vi "irrad calc lumens.vi"(8 "error in (no error)":errorcluster, 10 "IRRAD Input Parameters":T1, 11 "Color Parameters in":T2) -> (0 "error out":errorcluster, 2 "IRRAD Input Parameters out":T1, 3 "Color Parameters out":T2)   [LabVIEW 2013, in "AvaSpec.lvlib" / "AVSirrad_support.lvlib"]
uses:
  AVSirrad_support.lvlib
  Acquisition/AvaSpec Color Parameters.ctl
  Acquisition/Sphere Indicator.ctl
  IRRAD input parameters.ctl
  Libraries/IRRAD-DLL/AVSirrad.lvlib
  AvaSpec.lvlib
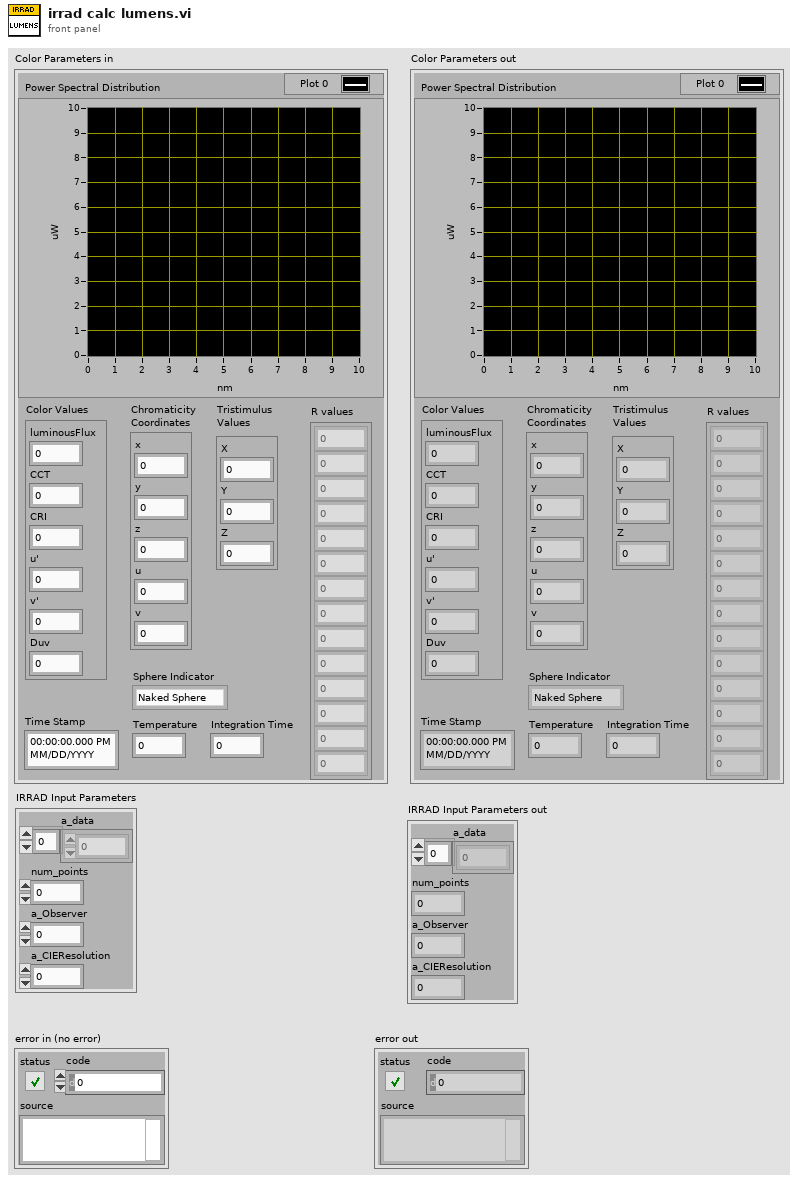
[diagram p1: front panel]
types:
  T1 = typedef "IRRAD input parameters.ctl" = cluster{"a_data":dbl[], "num_points":i32, "a_Observer":u8, "a_CIEResolution":u8}
  T2 = typedef "AvaSpec.lvlib/AvaSpec Color Parameters.ctl" = cluster{"Power Spectral Distribution":cluster{"X":dbl, "Y":dbl}[], "Color Values":cluster{"luminousFlux":dbl, "CCT":dbl, "CRI":dbl, "u'":dbl, "v'":dbl, "Duv":dbl}, "R values":dbl[], "Chromaticity \nCoordinates":cluster{"x":dbl, "y":dbl, "z":dbl, "u":dbl, "v":dbl}, "Tristimulus \nValues":cluster{"X":dbl, "Y":dbl, "Z":dbl}, "Time Stamp":timestamp, "Temperature":dbl, "Integration Time":dbl, "Sphere Indicator":T3}
  T3 = typedef "AvaSpec.lvlib/Sphere Indicator.ctl" = enum16{"Naked Sphere", "Insulated Sphere"}
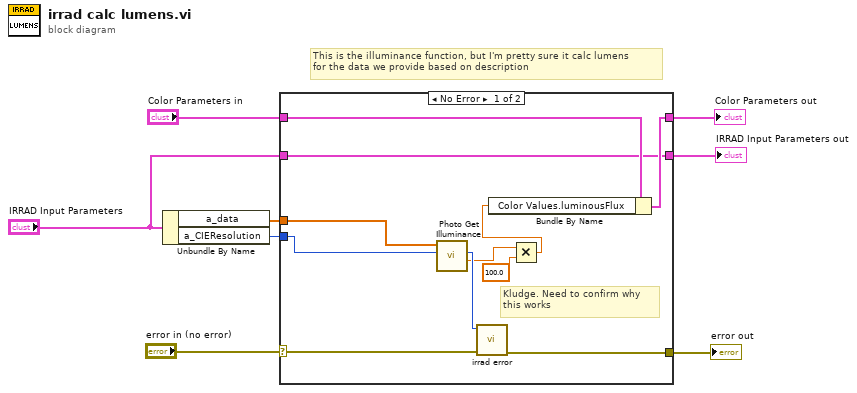
[diagram p0: block diagram]
diagram:
  # "This is the illuminance function, but I'm pretty sure it calc lumens \nfor the data we provide based on description"
  n1 = Unbundle By Name("IRRAD Input Parameters") -> ("a_data"=w4:dbl[], "a_CIEResolution"=w1:u8)
  n2 = case shown="No Error" "error in (no error)" {
    selector: "error in (no error)" -> [w19 w22]
    tunnel: [w18 w22] -> w7
    tunnel: w1 -> [w13 _]
    tunnel: "Color Parameters in" -> [w17 w21]
    tunnel: [w16 w21] -> w5
    tunnel: w4 -> [w14 _]
    tunnel: "IRRAD Input Parameters" -> [w15 w20]
    tunnel: [w15 w20] -> w2
    frame No Error {
      # "Kludge. Need to confirm why\nthis works"
      n3 = call "Photo Get Illuminance.vi"("a_CIEResolution"=w13, "a_data"=w14) -> ("a_Lux out"=w11:dbl, "function return"=w12:i16)  [unwired: 6 in, 2 out]
      n4 = call "irrad error.vi"("error in (no error)"=w19, "Output Value"=w12) -> ("error out"=w18:errorcluster)  [unwired: 9 in]
      n5 = Multiply(x=w11, y=100.0) -> (x*y=w9:dbl)
      n6 = Bundle By Name(cluster=w17, "Color Values.luminousFlux"=w9) -> (w16:T2)
    }
    frame Error {
    }
  }
  "error out" <- w7
  "Color Parameters out" <- w5
  "IRRAD Input Parameters out" <- w2
